vi "一致性检测VI.vi"(0 "位置范围设定":T8={"位置1"={"上限"=726.0, "下限"=686.0}, "位置2"={"上限"=874.0, "下限"=834.0}, "位置3"={"上限"=997.0, "下限"=957.0}, "位置4"={"上限"=1139.0, "下限"=1099.0}, "位置5"={"上限"=1283.0, "下限"=1243.0}, "位置6"={"上限"=1429.0, "下限"=1389.0}, "位置7"={"上限"=1576.0, "下限"=1536.0}, "位置8"={"上限"=1728.0, "下限"=1688.0}, "位置9"={"上限"=1879.0, "下限"=1839.0}, "位置10"={"上限"=2036.0, "下限"=1996.0}}, 1 "Image in":T1(plugin-control), 5 "导丝上料一致性参数":T7={"Rectangle"={"Left"=0, "Top"=0, "Right"=0, "Bottom"=0, "Rotation"=0.0}, "Find Straight Edge 1"={"Number of Lines"=1, "Type"=enum."First Edge Rake", "Min. Score"=10.0, "Max. Score"=1000.0, "Orientation"=0.0, "Angle Range"=45.0, "Angle Tolerance"=1.0, "Step Size"=11, "Min. SNR (db)"=0.0, "Min. Points (%)"=25.0, "Hough Iterations"=5}, "Process (Edge Detector 1)"=enum."Get All Edges", "Edge Options (Edge Detector 1)"={"Edge Polarity"=0, "Kernel Size"=9, "Width"=1, "Minimum Edge Strength"=8.0, "Interpolation Type"=enum."Bilinear Fixed", "Data Processing Method"=enum."Average"}, "Options (Find Straight Edge 1)"={"Search Direction"=0, "Edge Options"={"Edge Polarity"=0, "Kernel Size"=3, "Width"=1, "Minimum Edge Strength"=32.0, "Interpolation Type"=enum."Bilinear Fixed", "Data Processing Method"=enum."Average"}, "Show Search Area"=TRUE, "Show Search Lines"=TRUE, "Show Edges Found"=TRUE, "Show Result"=TRUE, "Search Area Color"=65280, "Search Lines Color"=255, "Edge Locations Color"=16776960, "Result Color"=16711680, "Overlay Group Name"=""}, "Parameters (Pattern Matching 1)"={"Number of Matches Requested"=1, "Minimum Match Score"=799.0, "Angle Ranges"=[{"Start Angle"=-180.0, "End Angle"=180.0}, {"Start Angle"=0.0, "End Angle"=360.0}]}, "Template File Path (Pattern Matching 1)"=path "D:/Inspect System/Source Code/Template Program/一致性模板.png"} {"Options (Find Straight Edge 1)"."Search Direction" items=["Left to Right", "Right to Left", "Top to Bottom", "Bottom to Top"]; "Options (Find Straight Edge 1)"."Edge Options"."Edge Polarity" items=["All Edges", "Rising Edges", "Falling Edges"]; "Options (Find Straight Edge 1)"."Edge Options"."Minimum Edge Strength" format="%.2f"; "Options (Find Straight Edge 1)"."Edge Options"."Width" step=2; "Options (Find Straight Edge 1)"."Edge Options"."Kernel Size" step=2; "Edge Options (Edge Detector 1)"."Edge Polarity" items=["All Edges", "Rising Edges", "Falling Edges"]; "Find Straight Edge 1"."Min. Points (%)" min=0.0 max=100.0; "Find Straight Edge 1"."Min. SNR (db)" min=0.0; "Find Straight Edge 1"."Max. Score" min=0.0 max=1024.0; "Find Straight Edge 1"."Min. Score" min=0.0 max=1024.0 step=1.0; "Rectangle"."Rotation" format="%.2f"; "Rectangle"."Left" scale=0.0..1024.0; "Rectangle"."Right" scale=0.0..1024.0}, 11 "error in (no error)":errorcluster caption="错误输入（无错误）") -> (3 "Image out":T1(plugin-control), 4 "位置坐标":sgl, 6 "基准边X坐标":sgl, 8 "字符串":string, 10 "数组":bool[](array[boolean]), 14 "动态范围":sgl[](array[numeric]), 15 "error out":errorcluster caption="错误输出")   [LabVIEW 2017]
uses:
  <vilib>/vision/Measure.llb/Edge New.ctl
  <vilib>/vision/Measure.llb/Straight Edge Options.ctl
  <vilib>/vision/Measure.llb/Straight Edge Process.ctl
  <vilib>/vision/Measure.llb/Edge Options.ctl
  <vilib>/vision/Measure.llb/Edge Polarity.ctl
panel:
  out "数组 3":sgl[][](array[numeric])
  out "x-y":sgl
  out "数组 2":i16[](array[numeric])
  out "Straight Edge (Find Straight Edge 1)":T9 {"Point2 (Real-World)"."Y" format="%.2f"; "Point2 (Real-World)"."X" format="%.2f"; "Point1 (Real-World)"."Y" format="%.2f"; "Point1 (Real-World)"."X" format="%.2f"; "Point2 (Pixels)"."Y" format="%.2f"; "Point2 (Pixels)"."X" format="%.2f"; "Point1 (Pixels)"."Y" format="%.2f"; "Point1 (Pixels)"."X" format="%.2f"}
  out "Edge Information (Edge Detector 1)":T10[](array[typedef]) {"Distance (Real-World)" format="%.2f"; "Location (Real-World)"."Y" format="%.2g"; "Location (Real-World)"."X" format="%.2f"; "Noise" format="%.2f"; "Location (Pixel)"."Y" format="%.2g"; "Location (Pixel)"."X" format="%.2f"; "Strength" format="%.2f"; "Distance (Pixel)" format="%.2f"}
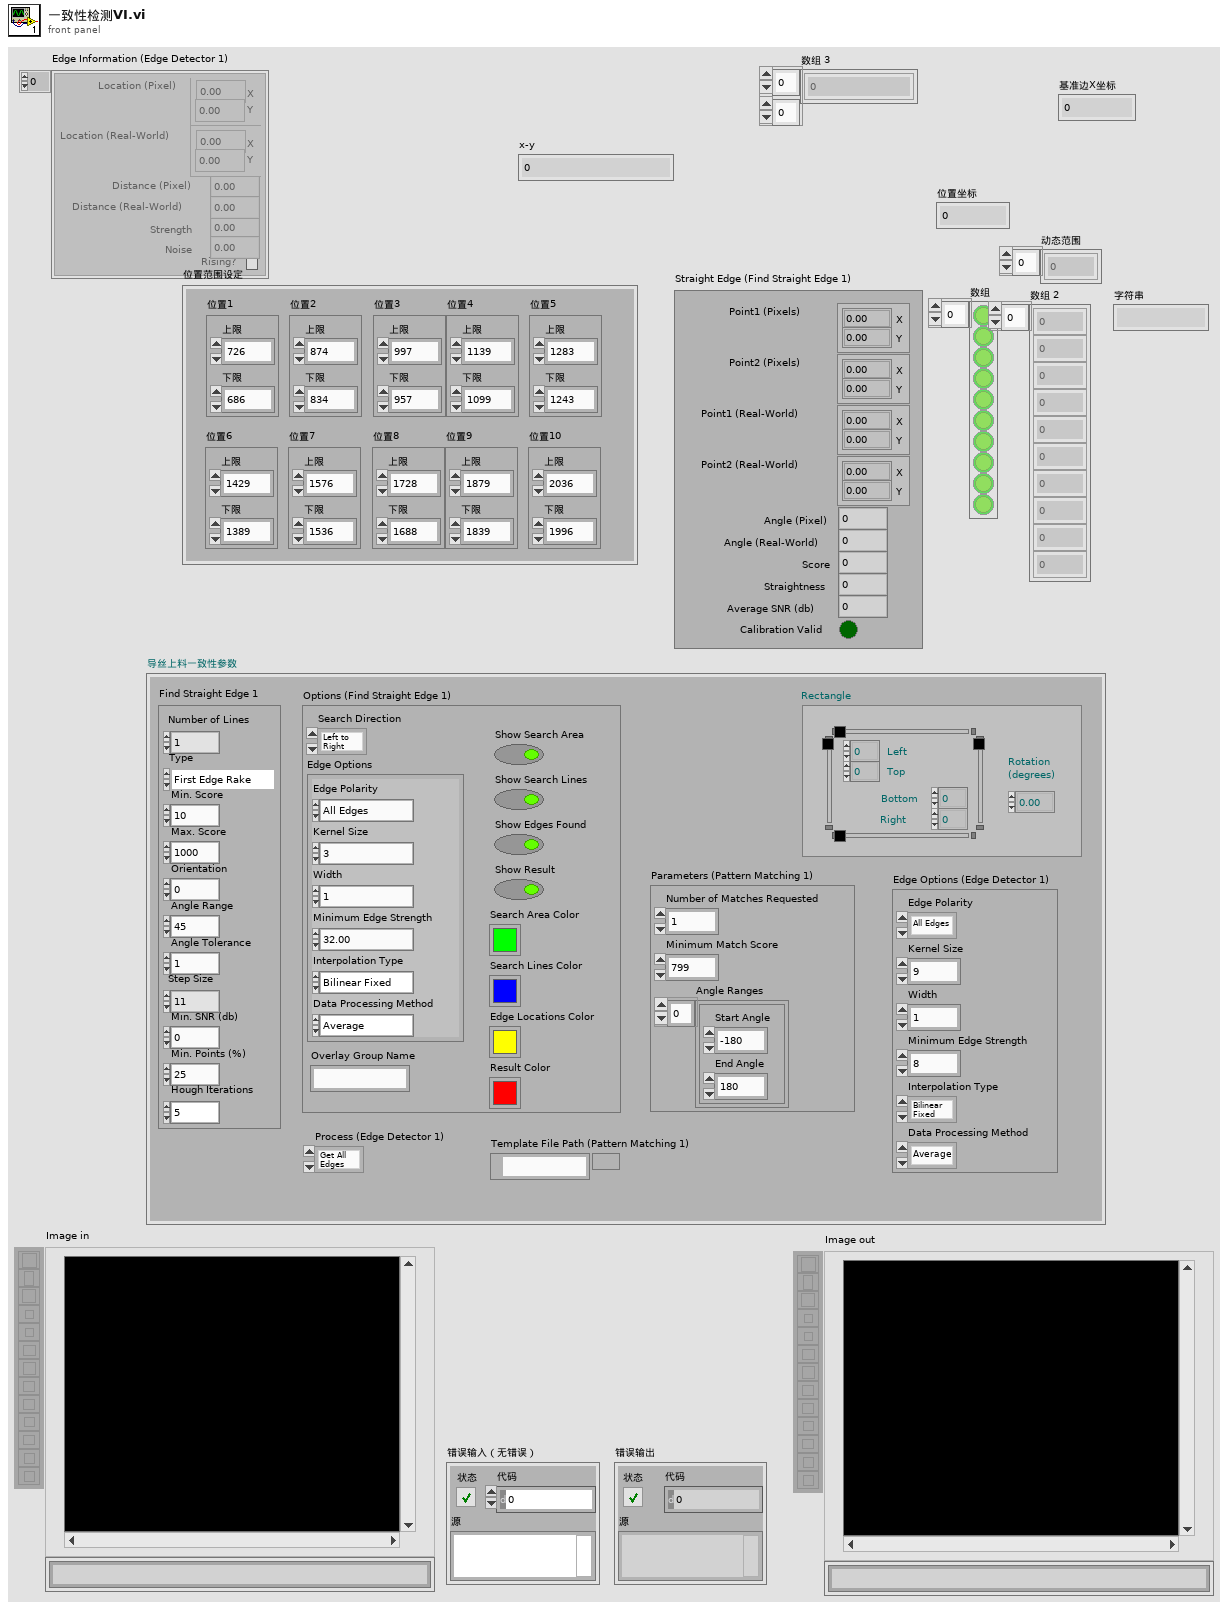
[diagram p1: front panel]
types:
  T1 = typedef "IMAQ Image.ctl" = refnum<image>
  T2 = typedef "IMAQ Rectangle" = cluster{"Left":i32, "Top":i32, "Right":i32, "Bottom":i32, "Rotation":dbl}
  T3 = typedef "Straight Edge Options.ctl" = cluster{"Number of Lines":i32, "Type":T4, "Min. Score":dbl, "Max. Score":dbl, "Orientation":dbl, "Angle Range":dbl, "Angle Tolerance":dbl, "Step Size":u32, "Min. SNR (db)":dbl, "Min. Points (%)":dbl, "Hough Iterations":i32}
  T4 = typedef "Straight Edge Process.ctl" = enum32{"First Edge Rake", "Best Edge Rake", "Hough Edge Rake", "First Edge Projection", "Best Edge Projection"}
  T5 = typedef "Edge Options.ctl" = cluster{"Edge Polarity":T6, "Kernel Size":u32, "Width":u32, "Minimum Edge Strength":sgl, "Interpolation Type":enum32{"Zero Order", "Bilinear", "Quadratic", "Cubic", "Bilinear Fixed"}, "Data Processing Method":enum32{"Average", "Median"}}
  T6 = typedef "Edge Polarity.ctl" = u32
  T7 = cluster{"Rectangle":T2, "Find Straight Edge 1":T3, "Process (Edge Detector 1)":enum16{"Get First Edge", "Get First + Last Edge", "Get All Edges", "Get Best Edge"}, "Edge Options (Edge Detector 1)":cluster{"Edge Polarity":u32, "Kernel Size":u32, "Width":u32, "Minimum Edge Strength":sgl, "Interpolation Type":enum32{"Zero Order", "Bilinear", "Quadratic", "Cubic", "Bilinear Fixed"}, "Data Processing Method":enum32{"Average", "Median"}}, "Options (Find Straight Edge 1)":cluster{"Search Direction":u32, "Edge Options":T5, "Show Search Area":bool, "Show Search Lines":bool, "Show Edges Found":bool, "Show Result":bool, "Search Area Color":u32, "Search Lines Color":u32, "Edge Locations Color":u32, "Result Color":u32, "Overlay Group Name":string}, "Parameters (Pattern Matching 1)":cluster{"Number of Matches Requested":i32, "Minimum Match Score":sgl, "Angle Ranges":cluster{"Start Angle":sgl, "End Angle":sgl}[]}, "Template File Path (Pattern Matching 1)":path}
  T8 = cluster{"位置1":cluster{"上限":dbl, "下限":dbl}, "位置2":cluster{"上限":dbl, "下限":dbl}, "位置3":cluster{"上限":dbl, "下限":dbl}, "位置4":cluster{"上限":dbl, "下限":dbl}, "位置5":cluster{"上限":dbl, "下限":dbl}, "位置6":cluster{"上限":dbl, "下限":dbl}, "位置7":cluster{"上限":dbl, "下限":dbl}, "位置8":cluster{"上限":dbl, "下限":dbl}, "位置9":cluster{"上限":dbl, "下限":dbl}, "位置10":cluster{"上限":dbl, "下限":dbl}}
  T9 = cluster{"Point1 (Pixels)":cluster{"X":sgl, "Y":sgl}, "Point2 (Pixels)":cluster{"X":sgl, "Y":sgl}, "Point1 (Real-World)":cluster{"X":sgl, "Y":sgl}, "Point2 (Real-World)":cluster{"X":sgl, "Y":sgl}, "Angle (Pixel)":dbl, "Angle (Real-World)":dbl, "Score":dbl, "Straightness":dbl, "Average SNR (db)":dbl, "Calibration Valid":bool}
  T10 = typedef "Edge New.ctl" = cluster{"Location (Pixel)":cluster{"X":sgl, "Y":sgl}, "Location (Real-World)":cluster{"X":sgl, "Y":sgl}, "Distance (Pixel)":dbl, "Distance (Real-World)":dbl, "Strength":dbl, "Noise":dbl, "Rising?":bool}
  T11 = enum16{"Get First Edge", "Get First + Last Edge", "Get All Edges", "Get Best Edge"}
  T12 = cluster{"Edge Polarity":u32, "Kernel Size":u32, "Width":u32, "Minimum Edge Strength":sgl, "Interpolation Type":enum32{"Zero Order", "Bilinear", "Quadratic", "Cubic", "Bilinear Fixed"}, "Data Processing Method":enum32{"Average", "Median"}}
  T13 = cluster{"Search Direction":u32, "Edge Options":T5, "Show Search Area":bool, "Show Search Lines":bool, "Show Edges Found":bool, "Show Result":bool, "Search Area Color":u32, "Search Lines Color":u32, "Edge Locations Color":u32, "Result Color":u32, "Overlay Group Name":string}
  T14 = cluster{"Number of Matches Requested":i32, "Minimum Match Score":sgl, "Angle Ranges":cluster{"Start Angle":sgl, "End Angle":sgl}[]}
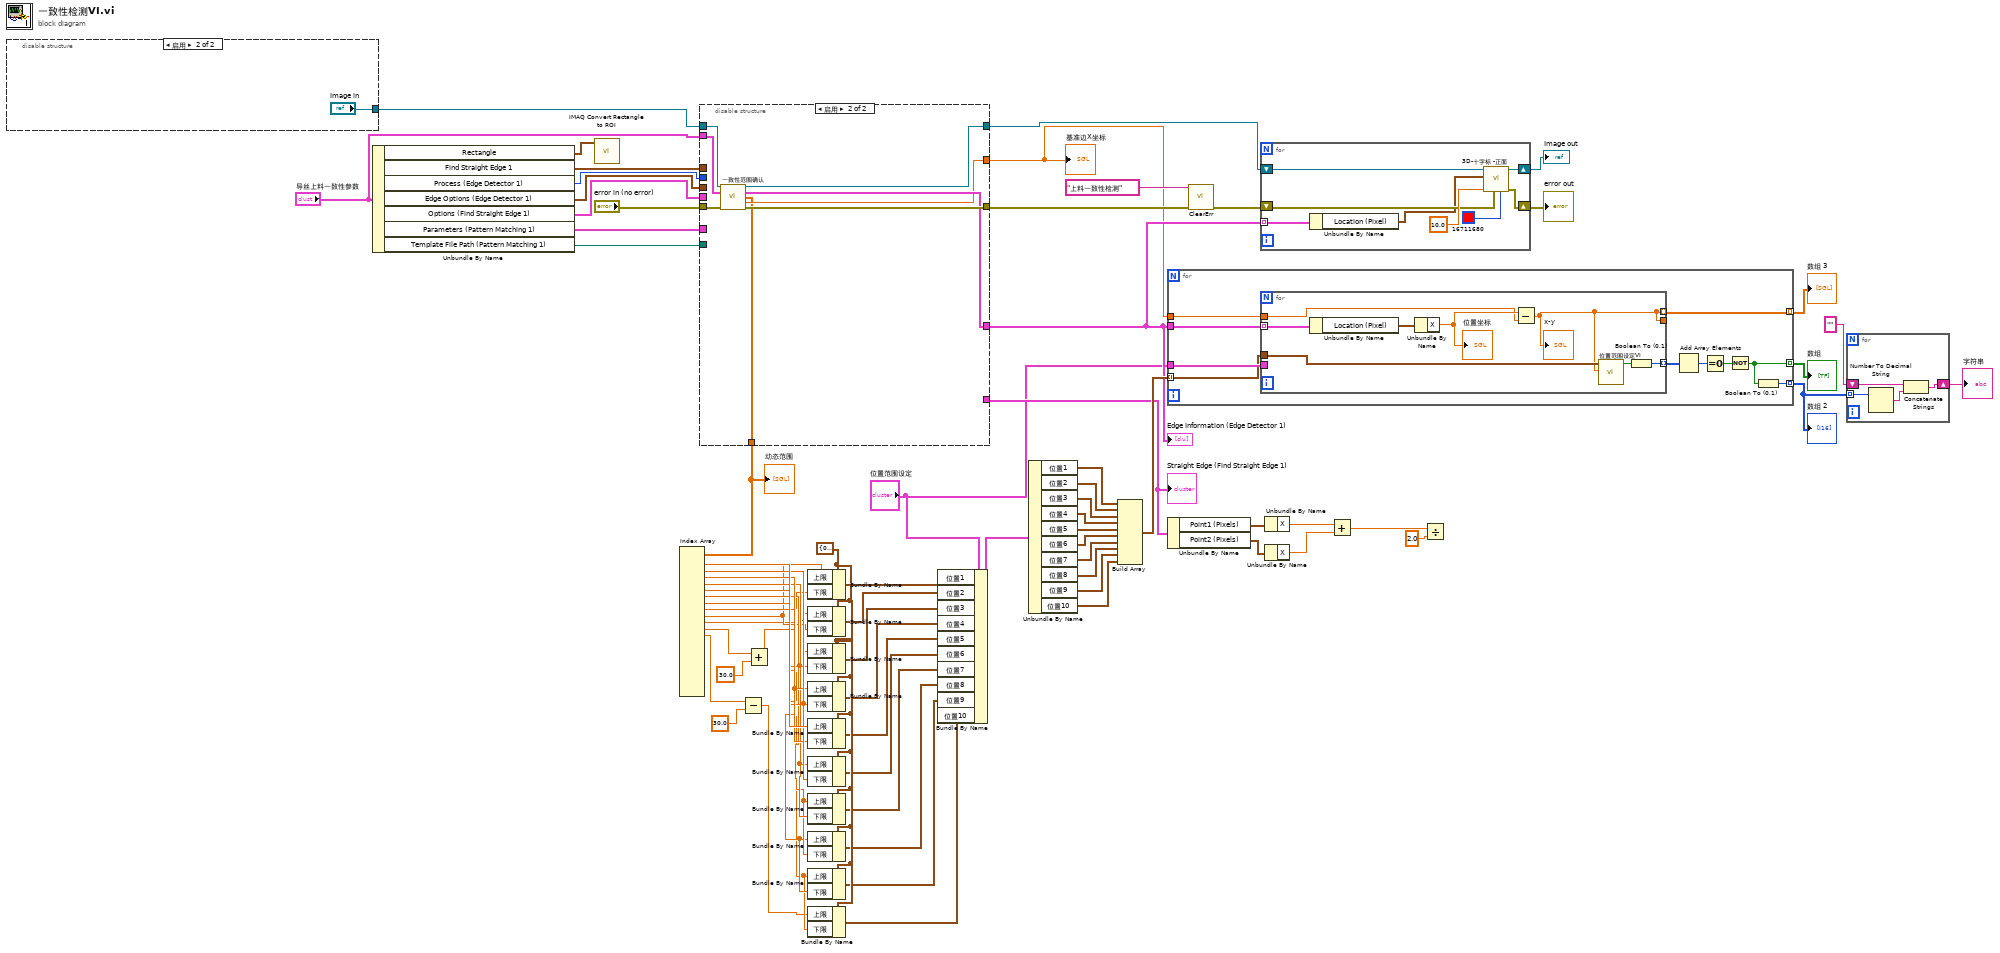
[diagram p0: block diagram]
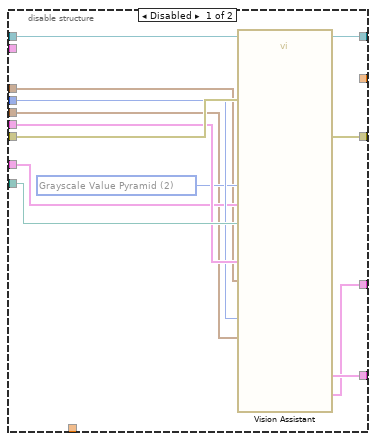
[diagram p2: hidden frame]
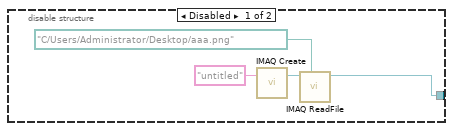
[diagram p3: hidden frame]
diagram:
  w27 = cluster{"上限":dbl, "下限":dbl} {"上限"=0.0, "下限"=0.0} ("位置1")
  n1 = disable-structure shown="启用" {
    disable-tunnel: [w73 "Image in"] -> w71
    frame Disabled {
      n2 = call "IMAQ Create"("Image Name"="untitled") -> ("New Image"=w75:T1)  [unwired: 4 in, 1 out]
      n3 = call "IMAQ ReadFile"("File Path"=path "C:/Users/Administrator/Desktop/aaa.png", "Image"=w75) -> ("Image Out"=w73:T1)  [unwired: 5 in, 4 out]
    }
    frame Enabled {
    }
  }
  n4 = Unbundle By Name("导丝上料一致性参数") -> ("Rectangle"=w34:T2, "Find Straight Edge 1"=w39:T3, "Process (Edge Detector 1)"=w41:T11, "Edge Options (Edge Detector 1)"=w38:T12, "Options (Find Straight Edge 1)"=w42:T13, "Parameters (Pattern Matching 1)"=w40:T14, "Template File Path (Pattern Matching 1)"=w43:path)
  n5 = call "IMAQ Convert Rectangle to ROI"("Rectangle"=w34) -> ()  [unwired: 8 in, 2 out]
  n6 = disable-structure shown="启用" {
    disable-tunnel: w71 -> [w89 w94]
    disable-tunnel: "error in (no error)" -> [w88 w97]
    disable-tunnel: [w87 _] -> w48
    disable-tunnel: [w86 w95] -> w47
    disable-tunnel: [w85 w92] -> w44
    disable-tunnel: w43 -> [w84 _]
    disable-tunnel: w42 -> [w83 _]
    disable-tunnel: w41 -> [w82 _]
    disable-tunnel: w40 -> [w81 _]
    disable-tunnel: w39 -> [w79 _]
    disable-tunnel: w38 -> [w78 _]
    disable-tunnel: [w77 w96] -> w37
    disable-tunnel: "导丝上料一致性参数" -> [_ w93]
    disable-tunnel: [_ w91] -> w31
    disable-tunnel: [_ w90] -> w30
    frame Disabled {
      w80 = 2 items=["All", "Low Discrepancy Sampling", "Grayscale Value Pyramid", "Gradients Pyramid"] ("Algorithm (Pattern Matching 1)")
      n7 = call "Vision Assistant"("Image In"=w89, "Options (Find Straight Edge 1)"=w83, "Fit Options (Find Straight Edge 1)"=w79, "Process (Edge Detector 1)"=w82, "error in"=w88, "Edge Options (Edge Detector 1)"=w78, "Algorithm (Pattern Matching 1)"=w80, "Parameters (Pattern Matching 1)"=w81, "Template File Path (Pattern Matching 1)"=w84) -> ("Image Out"=w86:T1, "Edge Information (Edge Detector 1)"=w85:T10[], "Straight Edge (Find Straight Edge 1)"=w87:T9, "error out"=w77:errorcluster)  [unwired: 14 in, 1 out]
    }
    frame Enabled {
      n8 = call "一致性范围确认.vi"("Image in"=w94, "导丝上料一致性参数"=w93, "error in (no error)"=w97) -> ("Image out"=w95:T1, "Edge Information (Edge Detector 1)"=w92:T10[], "动态范围"=w90:sgl[], "start X"=w91:sgl, "error out"=w96:errorcluster)  [unwired: 8 in]
    }
  }
  "Edge Information (Edge Detector 1)" <- w44
  "Straight Edge (Find Straight Edge 1)" <- w48
  "基准边X坐标" <- w31
  "动态范围" <- w30
  n9 = Index Array(array=w30) -> (element #1=w17:sgl, element #2=w16:sgl, element #3=w15:sgl, element #4=w14:sgl, element #5=w13:sgl, element #6=w12:sgl, element #7=w11:sgl, element #8=w10:sgl, element #9=w9:sgl, element #10=w7:sgl, element #11=w8:sgl, element #12=w2:sgl)  [unwired: 21 in, 9 out]
  n10 = Subtract(x=w2, y=sgl 30.0) -> (x-y=w1:sgl)
  n11 = Add(x=w8, y=sgl 30.0) -> (x+y=w5:sgl)
  n12 = Bundle By Name(cluster=w27, "上限"=w9, "下限"=w5) -> (w28:cluster{"上限":dbl, "下限":dbl})
  n13 = Bundle By Name(cluster=w27, "上限"=w11, "下限"=w9) -> (w26:cluster{"上限":dbl, "下限":dbl})
  n14 = Bundle By Name(cluster=w27, "上限"=w13, "下限"=w11) -> (w25:cluster{"上限":dbl, "下限":dbl})
  n15 = Bundle By Name(cluster=w27, "上限"=w15, "下限"=w13) -> (w24:cluster{"上限":dbl, "下限":dbl})
  n16 = Bundle By Name(cluster=w27, "上限"=w17, "下限"=w15) -> (w23:cluster{"上限":dbl, "下限":dbl})
  n17 = Bundle By Name(cluster=w27, "上限"=w14, "下限"=w16) -> (w22:cluster{"上限":dbl, "下限":dbl})
  n18 = Bundle By Name(cluster=w27, "上限"=w12, "下限"=w14) -> (w21:cluster{"上限":dbl, "下限":dbl})
  n19 = Bundle By Name(cluster=w27, "上限"=w10, "下限"=w12) -> (w20:cluster{"上限":dbl, "下限":dbl})
  n20 = Bundle By Name(cluster=w27, "上限"=w7, "下限"=w10) -> (w19:cluster{"上限":dbl, "下限":dbl})
  n21 = Bundle By Name(cluster=w27, "上限"=w1, "下限"=w7) -> (w18:cluster{"上限":dbl, "下限":dbl})
  n22 = Bundle By Name(cluster="位置范围设定", "位置1"=w28, "位置2"=w26, "位置3"=w25, "位置4"=w24, "位置5"=w23, "位置6"=w22, "位置7"=w21, "位置8"=w20, "位置9"=w19, "位置10"=w18) -> (w6:T8)
  n23 = Unbundle By Name(w6) -> ("位置1"=w64:cluster{"上限":dbl, "下限":dbl}, "位置2"=w63:cluster{"上限":dbl, "下限":dbl}, "位置3"=w62:cluster{"上限":dbl, "下限":dbl}, "位置4"=w61:cluster{"上限":dbl, "下限":dbl}, "位置5"=w60:cluster{"上限":dbl, "下限":dbl}, "位置6"=w59:cluster{"上限":dbl, "下限":dbl}, "位置7"=w58:cluster{"上限":dbl, "下限":dbl}, "位置8"=w57:cluster{"上限":dbl, "下限":dbl}, "位置9"=w56:cluster{"上限":dbl, "下限":dbl}, "位置10"=w55:cluster{"上限":dbl, "下限":dbl})
  n24 = Build Array(w64, w63, w62, w61, w60, w59, w58, w57, w56, w55) -> (w54:cluster{"上限":dbl, "下限":dbl}[])
  n25 = for {
    tunnel: w44 -> [w107]
    tunnel: "位置范围设定" -> [w106]
    tunnel: w54 -> [w105] mode=indexing
    tunnel: [w101] -> w53 mode=indexing
    tunnel: [w100] -> w52 mode=indexing
    tunnel: w31 -> [w99]
    tunnel: [w98] -> w33 mode=indexing
    n26 = for {
      tunnel: w107 -> [w115] mode=indexing
      tunnel: w106 -> [_]
      tunnel: w105 -> [w113]
      tunnel: [w111] -> w104 mode=indexing
      tunnel: w99 -> [w109]
      tunnel: [w108] -> _
      tunnel: [w108] -> w98 mode=indexing
      n27 = Unbundle By Name(w115) -> ("Location (Pixel)"=w114:cluster{"X":sgl, "Y":sgl})
      n28 = Unbundle By Name(w114) -> ("X"=w110:sgl)
      "位置坐标" <- w110
      n29 = Subtract(x=w110, y=w109) -> (x-y=w108:sgl)
      "x-y" <- w108
      n30 = call "位置范围设定VI.vi"("x"=w108, "位置1"=w113) -> ("1"=w112:bool)  [unwired: 9 in]
      n31 = Boolean To (0,1)(Boolean=w112) -> (0, 1=w111:i16)
    }
    n32 = Add Array Elements(numeric array=w104) -> (sum=w102:i16)
    n33 = Equal To 0?(x=w102) -> (x = 0?=w103:bool)
    n34 = Not(x=w103) -> (.not. x?=w101:bool)
    n35 = Boolean To (0,1)(Boolean=w101) -> (0, 1=w100:i16)
  }
  "数组" <- w53
  "数组 2" <- w52
  "数组 3" <- w33
  n36 = Unbundle By Name(w48) -> ("Point1 (Pixels)"=w70:cluster{"X":sgl, "Y":sgl}, "Point2 (Pixels)"=w69:cluster{"X":sgl, "Y":sgl})
  n37 = call "ClearErr.vi"("error in (no error)"=w37, "运行位置"="上料一致性检测") -> ("error out"=w36:errorcluster)  [unwired: 9 in]
  n38 = for {
    shift-right: [w120] -> w46
    shift-left: w47 -> [w123]
    shift-right: [w118] -> w45
    shift-left: w36 -> [w119]
    tunnel: w44 -> [w117] mode=indexing
    n39 = Unbundle By Name(w117) -> ("Location (Pixel)"=w116:cluster{"X":sgl, "Y":sgl})
    n40 = call "3D-十字标 -正面.vi"("Color"=u32 16711680, "error in (no error)"=w119, "radius"=10.0, "Target Point"=w116, "输入图片"=w123) -> ("error out"=w118:errorcluster, "输出图片"=w120:T1)  [unwired: 5 in]
  }
  "Image out" <- w46
  "error out" <- w45
  n41 = Unbundle By Name(w70) -> ("X"=w68:sgl)
  n42 = Unbundle By Name(w69) -> ("X"=w67:sgl)
  n43 = Add(x=w68, y=w67) -> (x+y=w66:sgl)
  n44 = Divide(x=w66, y=sgl 2.0) -> ()  [unwired: 1 out]
  n45 = for {
    tunnel: w52 -> [w127] mode=indexing
    shift-right: [w124] -> w50
    shift-left: "" -> [w126]
    n46 = Number To Decimal String(number=w127) -> (decimal integer string=w125:string)  [unwired: 1 in]
    n47 = Concatenate Strings(w126, w125) -> (w124:string)
  }
  "字符串" <- w50
